vi "RS232 close.vi"(1 "error in":errorcluster, 2 "VISA resource name in":refnum<visa-resource-name>) -> (0 "error out":errorcluster)   [LabVIEW 2014]
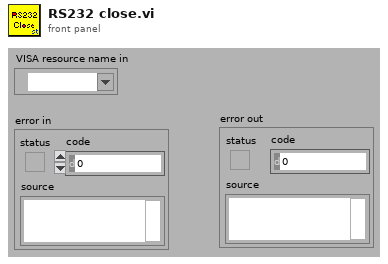
[diagram p1: front panel]
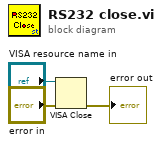
[diagram p0: block diagram]
diagram:
  n1 = VISA Close(VISA resource name="VISA resource name in", error in (no error)="error in") -> (error out=→"error out":errorcluster)
